vi "Aero_Chilled_Water_PID.vi"(1 "Present Value":dbl=15.0 format="%.2f", 2 "Previous Control Sum":dbl format="%.2f", 3 "Setpoint":dbl=15.0 format="%.2f") -> (0 "Dem Output":dbl format="%.2f")   [LabVIEW 2010]
uses:
  <vilib>/Analysis/NI_AALPro.lvlib
panel:
  in  "O/P deadband":dbl=1.0 format="%.2f"
  in  "Kp Deadband":dbl format="%.2f"
  in  "Derivative History":i32=6
  out "deadbanded error":dbl format="%.2f"
  in  "P":bool=TRUE
  in  "D":bool=TRUE
  in  "I":bool=TRUE
  out "Waveform Chart":T1(graph)
  in  "Manual Demand":dbl min=0.0 max=100.0 format="%.2f"
  in  "Manual Override":bool
  out "Control Sum":dbl format="%.2f"
  out "Derivative Term":dbl format="%.2f"
  out "Integral Term":dbl format="%.2f"
  out "error differential":dbl format="%.5f"
  out "error integral":dbl format="%.2f"
  out "Proportional Term":dbl format="%.2f"
  in  "Kd":dbl=4.0 format="%.2f"
  in  "Ki":dbl=15.0 format="%.2f"
  in  "Kp":dbl=12.0 format="%.2f"
  out "error":dbl format="%.2f"
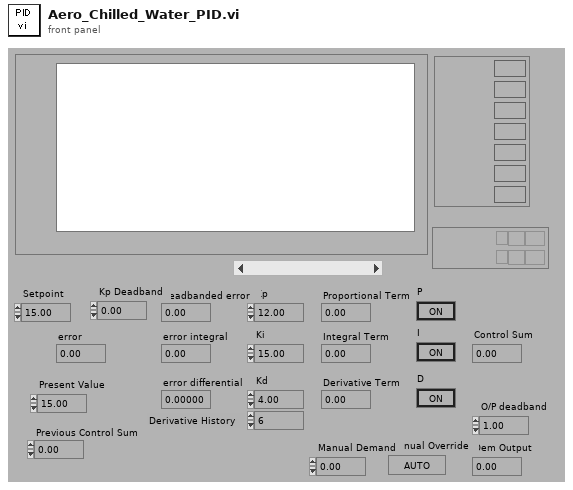
[diagram p1: front panel]
types:
  T1 = cluster{"Setpoint":dbl, "Present Value":dbl, "Proportional Term":dbl, "Integral Term":dbl, "Derivative Term":dbl, "Control Sum":dbl, "Dem Output":dbl}
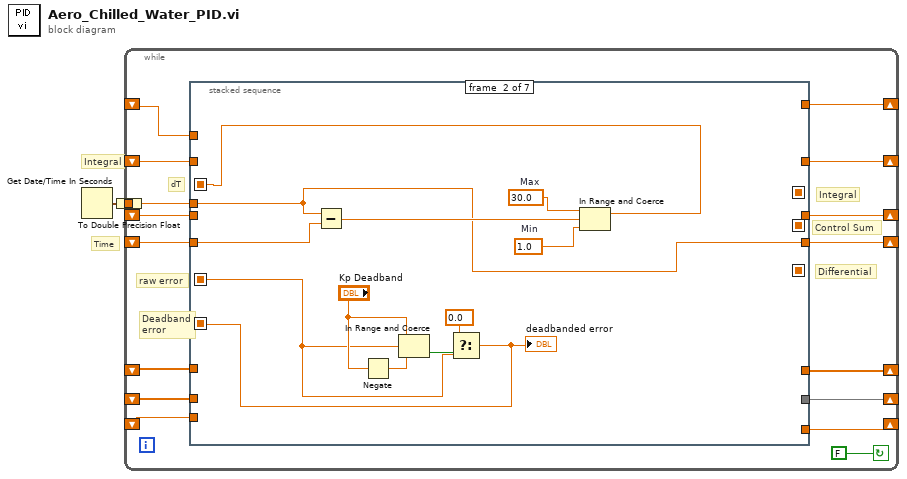
[diagram p0: block diagram]
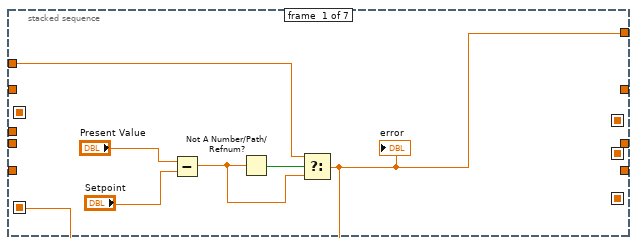
[diagram p2: hidden frame]
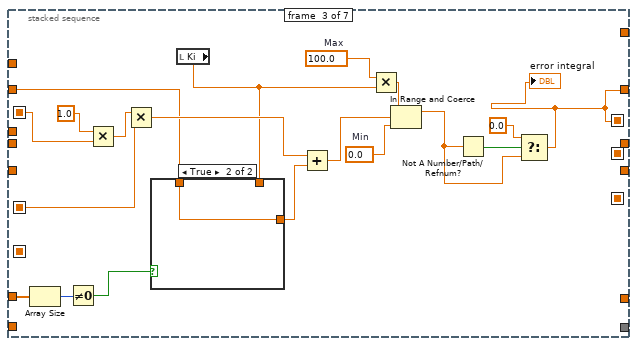
[diagram p3: hidden frame]
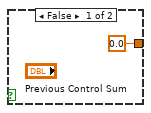
[diagram p4: hidden frame]
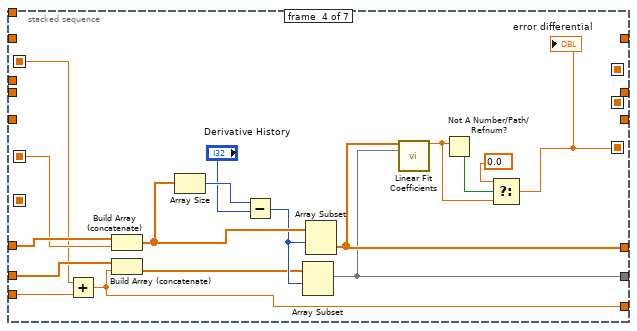
[diagram p5: hidden frame]
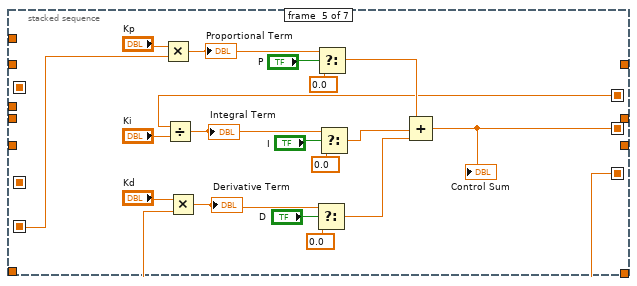
[diagram p6: hidden frame]
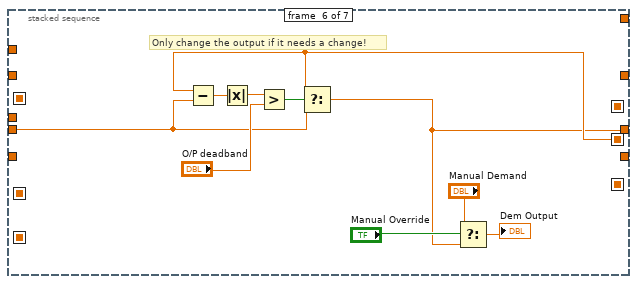
[diagram p7: hidden frame]
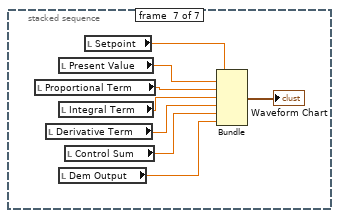
[diagram p8: hidden frame]
diagram:
  # "Integral"
  # "Time"
  n1 = Get Date/Time In Seconds() -> (seconds since 1Jan1904=w1:timestamp)
  n2 = To Double Precision Float(number=w1) -> (double precision float=w2:dbl)
  n3 = while {
    shift-left: _ -> [w5]
    shift-right: [w4] -> _
    shift-left: _ -> [w7]
    shift-right: [w6] -> _
    shift-left: _ -> [w9]
    shift-right: [w8] -> _
    tunnel: w2 -> [w14]
    shift-left: _ -> [w11]
    shift-right: [w10] -> _
    shift-left: _ -> [w13]
    shift-right: [w12] -> _
    shift-left: _ -> [w15]
    shift-right: [w16] -> _
    shift-left: _ -> [w18]
    shift-right: [w17] -> _
    stop <- FALSE continue-if-true
    # "Control Sum"
    # "raw error"
    # "Differential"
    # "Integral"
    # "Deadband\nerror"
    # "dT"
    n4 = stacked-sequence {
      seq-local: [_ w25 _ _ _ _ _] -> [_ _ w38 w60 _ _ _]
      seq-local: [_ w34 _ _ _ _ _] -> [_ _ _ _ w78 _ _]
      seq-local: [_ _ _ w65 _ _ _] -> [_ _ _ _ w77 _ _]
      seq-local: [_ _ w40 _ _ _ _] -> [_ _ _ _ w76 _ _]
      seq-local: [w19 _ _ _ _ _ _] -> [_ w26 w51 w66 _ _ _]
      seq-local: [_ _ _ _ w81 _ _] -> [_ _ _ _ _ w97 _]
      tunnel: w18 -> [_ w31 _ _ _ _ _]
      tunnel: [_ w29 _ _ _ _ _] -> w17
      tunnel: [_ _ w40 _ _ _ _] -> w16
      tunnel: w15 -> [_ _ w45 _ _ _ _]
      tunnel: w14 -> [_ w29 _ _ _ _ _]
      tunnel: w13 -> [_ _ w50 w74 _ _ _]
      tunnel: [_ _ _ w67 _ _ _] -> w12
      tunnel: w11 -> [_ _ _ w73 _ _ _]
      tunnel: [_ _ _ w64 _ _ _] -> w10
      tunnel: w9 -> [_ _ _ _ _ w95 _]
      tunnel: [_ _ _ _ _ w94 _] -> w8
      tunnel: w7 -> [_ _ _ w59 _ _ _]
      tunnel: [_ _ _ w58 _ _ _] -> w6
      tunnel: w5 -> [w21 _ _ _ _ _ _]
      tunnel: [w19 _ _ _ _ _ _] -> w4
      frame #0 {
        n5 = Subtract(x="Present Value", y="Setpoint") -> (x-y=w20:dbl)
        n6 = Not A Number/Path/Refnum?(number/path/refnum=w20) -> (NaN/Path/Refnum?=w22:bool)
        n7 = Select(t=w21, s=w22, f=w20) -> (s? t:f=w19:dbl)
        "error" <- w19
      }
      frame #1 {
        w32 = 1.0  # Min
        w33 = 30.0  # Max
        n8 = Subtract(x=w29, y=w31) -> (x-y=w30:dbl)
        n9 = Negate(x="Kp Deadband") -> (-x=w28:dbl)
        n10 = In Range and Coerce(upper limit="Kp Deadband", x=w26, lower limit=w28) -> (In Range?=w35:bool)  [unwired: 1 out]
        n11 = Select(t=0.0, s=w35, f=w26) -> (s? t:f=w34:dbl)
        "deadbanded error" <- w34
        n12 = In Range and Coerce(upper limit=w33, x=w30, lower limit=w32) -> (coerced(x)=w25:dbl)  [unwired: 1 out]
      }
      frame #2 {
        w55 = 0.0  # Min
        w54 = 100.0  # Max
        n13 = Array Size(array=w50) -> (size(s)=w49:i32)
        n14 = Not Equal To 0?(x=w49) -> (x != 0?=w47:bool)
        n15 = Multiply(x=1.0, y=w38) -> (x*y=w37:dbl)
        n16 = Multiply(x=w37, y=w51) -> (x*y=w48:dbl)
        n17 = local read "Ki"() -> (w44:dbl)
        n18 = case shown="True" w47 {
          tunnel: [0.0 ("Min") w57] -> w46
          tunnel: w45 -> [_ w57]
          tunnel: w44 -> [_ _]
          frame False {
          }
          frame True {
          }
        }
        n19 = Add(x=w48, y=w46) -> (x+y=w52:dbl)
        n20 = Multiply(x=w54, y=w44) -> (x*y=w53:dbl)
        n21 = In Range and Coerce(upper limit=w53, x=w52, lower limit=w55) -> (coerced(x)=w41:dbl)  [unwired: 1 out]
        n22 = Not A Number/Path/Refnum?(number/path/refnum=w41) -> (NaN/Path/Refnum?=w42:bool)
        n23 = Select(t=0.0, s=w42, f=w41) -> (s? t:f=w40:dbl)
        "error integral" <- w40
      }
      frame #3 {
        n24 = Add(x=w60, y=w59) -> (x+y=w58:dbl)
        n25 = Build Array (concatenate)(w74, w66) -> (w70:dbl[])
        n26 = Build Array (concatenate)(w73, w58) -> (w68:dbl[])
        n27 = Array Size(array=w70) -> (size(s)=w72:i32)
        n28 = Subtract(x=w72, y="Derivative History") -> (x-y=w69:i32)
        n29 = Array Subset(array=w68, index=w69) -> (w64:dbl[])  [unwired: 1 in]
        n30 = Array Subset(array=w70, index=w69) -> (w67:dbl[])  [unwired: 1 in]
        n31 = call <vilib>:"Linear Fit Coefficients.vi"("Y"=w67, "X"=w64) -> ("slope"=w61:dbl)  [unwired: 3 in, 10 out]
        n32 = Not A Number/Path/Refnum?(number/path/refnum=w61) -> (NaN/Path/Refnum?=w63:bool)
        n33 = Select(t=0.0 ("f"), s=w63, f=w61) -> (s? t:f=w65:dbl)
        "error differential" <- w65
      }
      frame #4 {
        n34 = Multiply(x="Kp", y=w78) -> (x*y=w91:dbl)
        "Proportional Term" <- w91
        n35 = Divide(x=w76, y="Ki") -> (x/y=w82:dbl)
        "Integral Term" <- w82
        n36 = Multiply(x="Kd", y=w77) -> (x*y=w83:dbl)
        "Derivative Term" <- w83
        n37 = Select(t=w83, s="D", f=0.0) -> (s? t:f=w85:dbl)
        n38 = Select(t=w91, s="P", f=0.0) -> (s? t:f=w92:dbl)
        n39 = Select(t=w82, s="I", f=0.0) -> (s? t:f=w84:dbl)
        n40 = Compound Arithmetic op=ADD(w92, w84, w85) -> (w81:dbl)
        "Control Sum" <- w81
      }
      frame #5 {
        # "Only change the output if it needs a change!"
        n41 = Subtract(x=w97, y=w95) -> (x-y=w100:dbl)
        n42 = Absolute Value(x=w100) -> (abs(x)=w99:dbl)
        n43 = Greater?(x=w99, y="O/P deadband") -> (0:w98:bool)
        n44 = Select(t=w97, s=w98, f=w95) -> (s? t:f=w94:dbl)
        n45 = Select(t="Manual Demand", s="Manual Override", f=w94) -> (s? t:f=→"Dem Output":dbl)
      }
      frame #6 {
        n46 = local read "Proportional Term"() -> (w107:dbl)
        n47 = local read "Derivative Term"() -> (w109:dbl)
        n48 = local read "Present Value"() -> (w106:dbl)
        n49 = local read "Integral Term"() -> (w108:dbl)
        n50 = local read "Dem Output"() -> (w111:dbl)
        n51 = local read "Control Sum"() -> (w110:dbl)
        n52 = local read "Setpoint"() -> (w105:dbl)
        n53 = Bundle("Setpoint"=w105, "Present Value"=w106, "Proportional Term"=w107, "Integral Term"=w108, "Derivative Term"=w109, "Control Sum"=w110, "Dem Output"=w111) -> (→"Waveform Chart":T1)  [unwired: 1 out]
      }
    }
  }
